vi "createSetForceFrame.vi"(0 "DAAILC in":refnum<class "DAAILC.lvclass">, 5 "WaitForTrigger":bool, 7 "TriggerIRQ":bool, 9 "SlewFlag":bool, 11 "error in (no error)":errorcluster) -> (4 "DAAILC out":refnum<class "DAAILC.lvclass">, 6 "Frame":T1 {"Data" format="%02x"}, 15 "error out":errorcluster)   [LabVIEW 2016, in "RTFAILC.lvlib" / "DAAILC.lvclass"]
uses:
  DAAILC.lvclass
  Common_RT_ILC/ILC/ILC.lvclass
  FAILC/FAILC.lvclass
  Common_RT_Modbus/DynamicFrameBuilder/DynamicFrameBuilder.lvclass
  D:/Code/Common_RT_FAILC/FAILC/FAILC.lvclass
  D:/Code/Common_RT_ILC/ILC/ILC.lvclass
  Common_RT_Modbus/DataTypes/Frame.ctl
  Common_RT_Modbus/RTModbus.lvlib
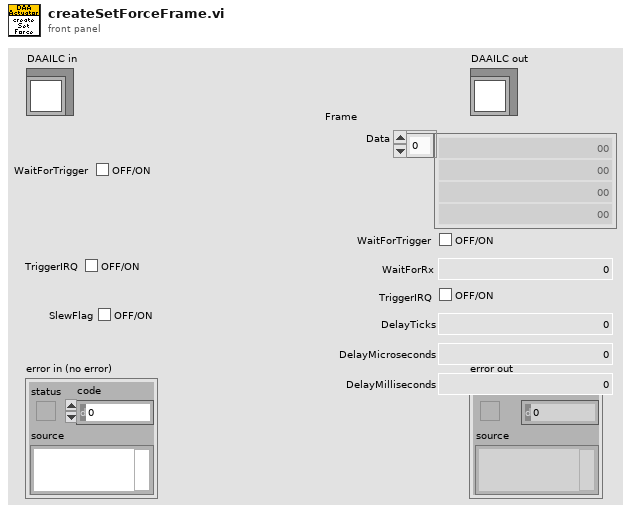
[diagram p1: front panel]
types:
  T1 = typedef "RTModbus.lvlib/Frame.ctl" = cluster{"Data":u8[], "WaitForTrigger":bool, "WaitForRx":u16, "TriggerIRQ":bool, "DelayTicks":u16, "DelayMicroseconds":u16, "DelayMilliseconds":u16}
  T2 = typedef "RTILC.lvlib/ILCData.ctl" = cluster{"Constants":T3, "Command":T4, "Telemetry":T6, "Responses":T7, "Timings":T9}
  T3 = typedef "RTILC.lvlib/ILCConstants.ctl" = cluster{"Subnet":u8, "Address":u8}
  T4 = typedef "RTILC.lvlib/ILCCommand.ctl" = cluster{"ILCMode":u16, "TemporaryAddress":u8, "ADCScanRate":T5, "ADCChannel":u8, "ADCOffset":sgl, "ADCSensitivity":sgl}
  T5 = typedef "RTILC.lvlib/ILCScanRates.ctl" = u8
  T6 = typedef "RTILC.lvlib/ILCTelemetry.ctl" = cluster{"UniqueID":u64, "FirmwareType":u8, "NetworkNodeType":u8, "ILCOption":u8, "NetworkNodeOption":u8, "MajorRevision":u8, "MinorRevision":u8, "FirmwareName":string, "ILCMode":u16, "MajorFault":bool, "MinorFault":bool, "FaultOverride":bool, "UniqueIDCRCMismatch":bool, "AppTypeNodeTypeMismatch":bool, "AppMissing":bool, "AppCRCMismatch":bool, "TEDSNotFound":bool, "TEDS1Mismatch":bool, "TEDS2Mismatch":bool, "WatchdogResetDetected":bool, "BrownoutDetected":bool, "EventTrapResetDetected":bool, "TemporaryAddress":u8, "ADCScanRate":T5, "DAC1":u16, "DAC2":u16, "DAC3":u16, "DAC4":u16, "MainADCCalibrationK":sgl[], "MainSensorOffset":sgl[], "MainSensorSensitivity":sgl[], "BackupADCCalibrationK":sgl[], "BackupSensorOffset":sgl[], "BackupSensorSensitivity":sgl[]}
  T7 = typedef "RTILC.lvlib/ILCResponses.ctl" = cluster{"ReportServerID":T8, "ReportServerStatus":T8, "ILCMode":T8, "SetTemporaryAddress":T8, "Reset":T8, "ADCScanRate":T8, "ADCOffsetSensitivity":T8, "ReadDAC":T8, "ReadCalibration":T8}
  T8 = typedef "RTModbus.lvlib/ExceptionCodes.ctl" = u16
  T9 = typedef "RTILC.lvlib/ILCTimings.ctl" = cluster{"ADCOffsetSensitivity":u32, "ADCScanRate":u32, "ILCMode":u32, "ReadCalibration":u32, "ReportServerID":u32, "ReportServerStatus":u32, "Reset":u32, "SetTemporaryAddress":u32}
  T10 = typedef "RTFAILC.lvlib/FAData.ctl" = cluster{"Constants":T11, "Command":T12, "Telemetry":T14, "Responses":T15, "Timings":T16}
  T11 = typedef "RTFAILC.lvlib/FAConstants.ctl" = cluster{"ID":i16}
  T12 = typedef "RTFAILC.lvlib/FACommand.ctl" = cluster{"AxialSetPoint":i32, "LateralSetPoint":i32, "PressureServoValveSettings":T13, "BoosterValveSettings":T13}
  T13 = typedef "RTFAILC.lvlib/FAPID.ctl" = cluster{"Kp":sgl, "Ki":sgl, "Kd":sgl, "Kf":sgl}
  T14 = typedef "RTFAILC.lvlib/FATelemetry.ctl" = cluster{"ILCFault":bool, "BroadcastCounter":u8, "AxialLoadCellForce":sgl, "LateralLoadCellForce":sgl, "AxialPressure":T13, "AxialTurbo":T13, "LateralPressure":T13, "LateralTurbo":T13}
  T15 = typedef "RTFAILC.lvlib/FAResponses.ctl" = cluster{"PIDParameters":T8, "ReadPIDParameters":T8, "SetForce":T8, "ForceAndStatus":T8}
  T16 = typedef "RTFAILC.lvlib/FATimings.ctl" = cluster{"BroadcastSetForce":u32, "PIDParameters":u32, "FreezeSensorValues":u32, "ForceAndStatus":u32, "ReadPIDParameters":u32, "SetForce":u32}
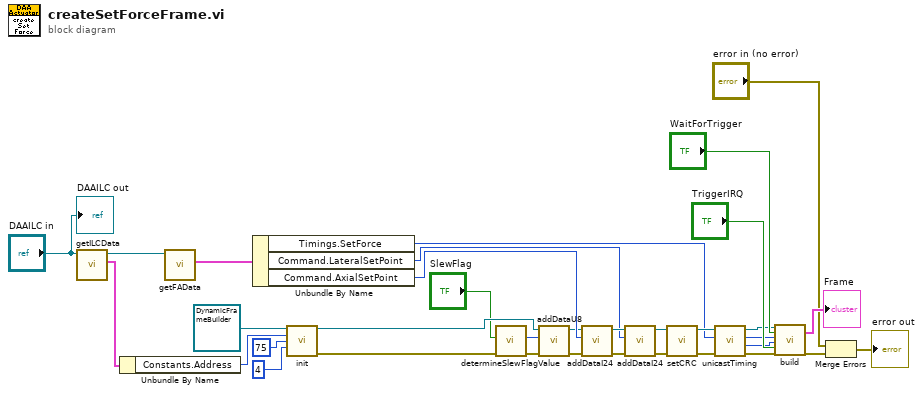
[diagram p0: block diagram]
diagram:
  n1 = call "getILCData.vi"("ILC in"="DAAILC in") -> ("ILCData"=w28:T2, "ILC out"=w29:refnum<class "DAAILC.lvclass">)  [unwired: 9 in]
  n2 = Unbundle By Name(w28) -> ("Constants.Address"=w34:u8)
  n3 = call "getFAData.vi"("FAILC in"=w29) -> ("FAData"=w27:T10)  [unwired: 9 in, 1 out]
  n4 = Unbundle By Name(w27) -> ("Timings.SetForce"=w3:u32, "Command.LateralSetPoint"=w17:i32, "Command.AxialSetPoint"=w19:i32)
  n5 = call "init.vi"("DynamicFrameBuilder in"=refnum<class "DynamicFrameBuilder.lvclass"> refnum ("RTModbus.lvlib:DynamicFrameBuilder.lvclass"), "Address"=w34, "Function"=u8 75, "DataSize"=4) -> ("DynamicFrameBuilder out"=w20:refnum<class "DynamicFrameBuilder.lvclass">, "error out"=w9:errorcluster)  [unwired: 10 in]
  n6 = call "determineSlewFlagValue.vi"("error in (no error)"=w9, "SlewFlag"="SlewFlag") -> ("error out"=w8:errorcluster, "FlagValue"=w10:u8)  [unwired: 7 in, 1 out]
  n7 = call "addDataU8.vi"("error in (no error)"=w8, "Data"=w10, "DynamicFrameBuilder in"=w20) -> ("error out"=w31:errorcluster, "DynamicFrameBuilder out"=w18:refnum<class "DynamicFrameBuilder.lvclass">)  [unwired: 7 in]
  n8 = call "addDataI24.vi"("error in (no error)"=w31, "Data"=w19, "DynamicFrameBuilder in"=w18) -> ("error out"=w26:errorcluster, "DynamicFrameBuilder out"=w25:refnum<class "DynamicFrameBuilder.lvclass">)  [unwired: 7 in]
  n9 = call "addDataI24.vi"("error in (no error)"=w26, "Data"=w17, "DynamicFrameBuilder in"=w25) -> ("error out"=w24:errorcluster, "DynamicFrameBuilder out"=w23:refnum<class "DynamicFrameBuilder.lvclass">)  [unwired: 7 in]
  n10 = call "setCRC.vi"("error in (no error)"=w24, "DynamicFrameBuilder in"=w23) -> ("error out"=w7:errorcluster, "DynamicFrameBuilder out"=w4:refnum<class "DynamicFrameBuilder.lvclass">)  [unwired: 8 in]
  n11 = call "unicastTiming.vi"("error in (no error)"=w7, "Latency in"=w3, "DynamicFrameBuilder in"=w4) -> ("error out"=w6:errorcluster, "WaitForRxTimeout"=w1:u16, "Latency out"=w2:u32, "DynamicFrameBuilder out"=w5:refnum<class "DynamicFrameBuilder.lvclass">)  [unwired: 5 in]
  n12 = call "build.vi"("DynamicFrameBuilder in"=w5, "WaitForTrigger"="WaitForTrigger", "Latency"=w2, "WaitForRxTimeout"=w1, "TriggerIRQ"="TriggerIRQ", "error in (no error)"=w6) -> ("Frame"=→"Frame":T1, "error out"=w30:errorcluster)  [unwired: 11 in, 1 out]
  n13 = Merge Errors("error in (no error)", w30) -> (→"error out":errorcluster)
  "DAAILC out" <- "DAAILC in"
